vi "Get Register Address Limit.vi"(8 "error in (no error)":errorcluster, 11 "RFFE Command in":refnum<class "RFFE Command.lvclass">) -> (0 "error out":errorcluster, 2 "Register Address Limit":T1 format="%02x", 3 "RFFE Command out":refnum<class "RFFE Command.lvclass">)   [LabVIEW 2018, in "MIPI RFFE API.lvlib" / "RFFE Command.lvclass"]
uses:
  RFFE Command.lvclass
  Register Address.ctl
  MIPI RFFE API.lvlib
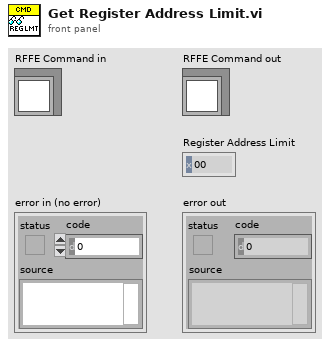
[diagram p1: front panel]
types:
  T1 = typedef "MIPI RFFE API.lvlib/Register Address.ctl" = u16
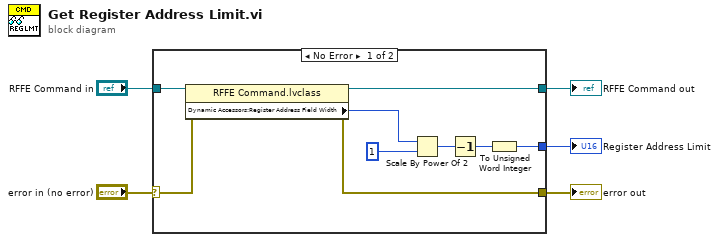
[diagram p0: block diagram]
diagram:
  n1 = case shown="No Error" "error in (no error)" {
    selector: "error in (no error)" -> [w8 w15]
    tunnel: "RFFE Command in" -> [w13 w16]
    tunnel: [w6 _] -> w1
    tunnel: [w9 w16] -> w4
    tunnel: [w7 w15] -> w2
    frame No Error {
      n2 = property class="RFFE Command.lvclass"(reference=w13, error in=w8) -> (reference out=w9:refnum<class "RFFE Command.lvclass">, error out=w7:errorcluster, "Dynamic Accessors:Register Address Field Width"=w12:i32)
      n3 = Scale By Power Of 2(n=w12, x=1) -> (x*2^n=w11:i32)
      n4 = Decrement(x=w11) -> (x-1=w10:i32)
      n5 = To Unsigned Word Integer(number=w10) -> (unsigned 16bit integer=w6:u16)
    }
    frame Error {
    }
  }
  "error out" <- w2
  "RFFE Command out" <- w4
  "Register Address Limit" <- w1
